vi "task6.vi"() -> ()   [LabVIEW 2017]
uses:
  5d7c750d-3047-46fd-b0c0-59bbbb6cc45c.vi
panel:
  out "Waveform Chart":u32(graph)
  in  "stop":bool
  out "Thermometer":dbl(slide) scale=0.0..255.0
  in  "Array":bool[](array[boolean])
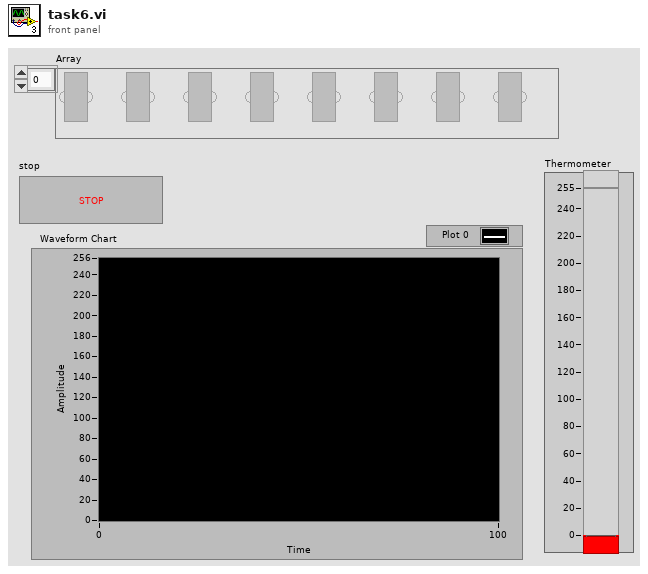
[diagram p1: front panel]
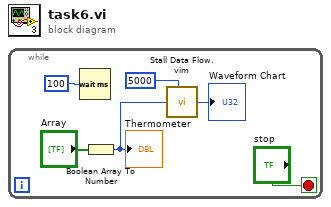
[diagram p0: block diagram]
diagram:
  n1 = while {
    stop <- "stop" stop-if-true
    n2 = Wait (ms)(milliseconds to wait=u32 100) -> ()  [unwired: 1 out]
    n3 = Boolean Array To Number(Boolean array="Array") -> (number=w3:u32)
    "Thermometer" <- w3
    n4 = call "Stall Data Flow.vim"("value in"=w3, "milliseconds to wait"=u32 5000) -> ("value out"=→"Waveform Chart":u32)  [unwired: 1 out]
  }
